vi "Create Temporary Database File.vi"(8 "error in (no error)":errorcluster) -> (0 "error out":errorcluster, 3 "path":path)   [LabVIEW 2020, in "Controller Test.lvclass"]
uses:
  Controller Test/Controller Test.lvclass
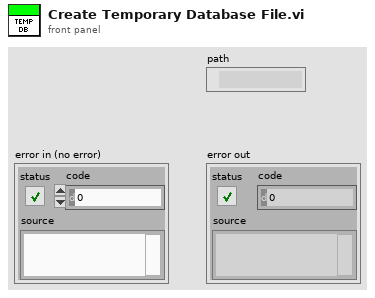
[diagram p1: front panel]
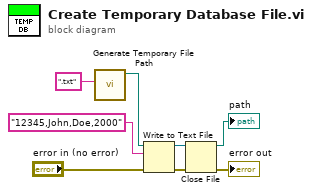
[diagram p0: block diagram]
diagram:
  n1 = call <vilib>:"Generate Temporary File Path.vi"("Temporary File Extension (tmp)"=".txt") -> ("Unique Temporary File Path"=w3:path)  [unwired: 9 in, 1 out]
  n2 = Write to Text File(file (use dialog)=w3, text="12345,John,Doe,2000", error in="error in (no error)") -> (refnum out=w5:refnum<file>, error out=w4:errorcluster)  [unwired: 1 in, 1 out]
  n3 = Close File(refnum=w5, error in=w4) -> (path=→"path":path, error out=→"error out":errorcluster)
